vi "case1(moveToShape).vi"(0 "Circles array":refnum<vi>, 1 "right-":refnum<vi>, 4 "defX":dbl, 5 "right+":refnum<vi>, 7 "left-":refnum<vi>, 8 "defY":sgl, 9 "x":refnum<vi>, 14 "left+":refnum<vi>, 15 "y":refnum<vi>, 16 "mainCase":refnum<vi>) -> (20 "Y":sgl, 21 "X":sgl)   [LabVIEW 2017]
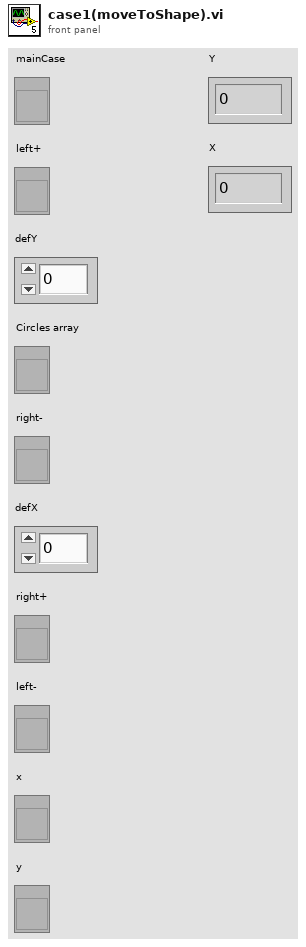
[diagram p1: front panel]
types:
  T1 = cluster{"Position":cluster{"X":sgl, "Y":sgl}, "Radius":dbl, "Score":dbl}[]
  T2 = cluster{"Position":cluster{"X":sgl, "Y":sgl}, "Radius":dbl, "Score":dbl}
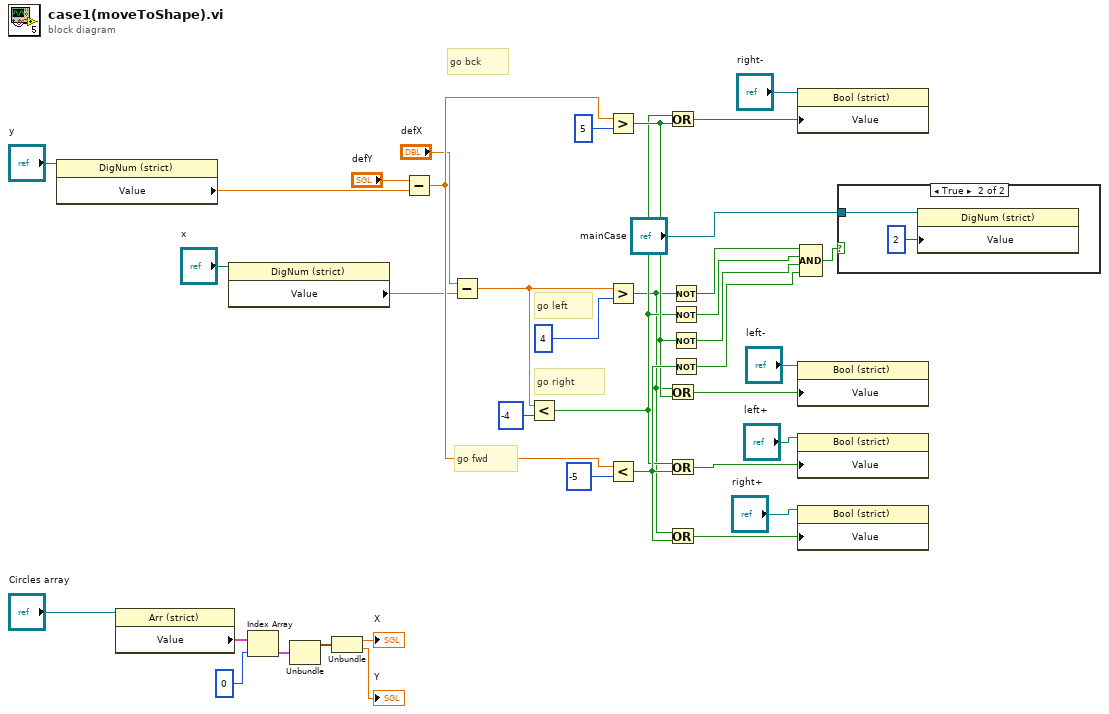
[diagram p0: block diagram]
diagram:
  # "go fwd"
  # "go bck"
  # "go right"
  # "go left"
  n1 = property class="DigNum (strict)"(reference="y") -> ("Value"=w23:sgl)  [unwired: 1 in, 2 out]
  n2 = property class="Arr (strict)"(reference="Circles array") -> ("Value"=w10:T1)  [unwired: 1 in, 2 out]
  n3 = property class="DigNum (strict)"(reference="x") -> ("Value"=w17:sgl)  [unwired: 1 in, 2 out]
  n4 = Index Array(array=w10, index=0) -> (element=w12:T2)
  n5 = Unbundle(w12) -> ("Position"=w13:cluster{"X":sgl, "Y":sgl})  [unwired: 2 out]
  n6 = Unbundle(w13) -> ("X"=→"X":sgl, "Y"=→"Y":sgl)
  n7 = Subtract(x="defY", y=w23) -> (x-y=w24:sgl)
  n8 = Subtract(x="defX", y=w17) -> (x-y=w27:dbl)
  n9 = Less?(x=w27, y=-4) -> (x < y?=w31:bool)
  n10 = Greater?(x=w24, y=5) -> (0:w32:bool)
  n11 = Greater?(x=w27, y=4) -> (0:w30:bool)
  n12 = Less?(x=w24, y=-5) -> (x < y?=w33:bool)
  n13 = Or(x=w31, y=w32) -> (x .or. y?=w18:bool)
  n14 = Or(x=w30, y=w32) -> (x .or. y?=w20:bool)
  n15 = Or(x=w31, y=w33) -> (x .or. y?=w21:bool)
  n16 = Or(x=w30, y=w33) -> (x .or. y?=w19:bool)
  n17 = Not(x=w30) -> (.not. x?=w34:bool)
  n18 = Not(x=w31) -> (.not. x?=w35:bool)
  n19 = Not(x=w32) -> (.not. x?=w36:bool)
  n20 = Not(x=w33) -> (.not. x?=w37:bool)
  n21 = property class="Bool (strict)"(reference="right-", "Value"=w18) -> ()  [unwired: 1 in, 2 out]
  n22 = property class="Bool (strict)"(reference="left-", "Value"=w20) -> ()  [unwired: 1 in, 2 out]
  n23 = property class="Bool (strict)"(reference="left+", "Value"=w21) -> ()  [unwired: 1 in, 2 out]
  n24 = property class="Bool (strict)"(reference="right+", "Value"=w19) -> ()  [unwired: 1 in, 2 out]
  n25 = Compound Arithmetic op=AND(w34, w35, w36, w37) -> (w1:bool)
  n26 = case shown="True" w1 {
    tunnel: "mainCase" -> [_ w38]
    frame False {
    }
    frame True {
      n27 = property class="DigNum (strict)"(reference=w38, "Value"=2 ("mainCase")) -> ()  [unwired: 1 in, 2 out]
    }
  }
